vi "dataValueToXml.vi"(8 "error in (no error)":errorcluster, 11 "RampEvent in":refnum<class "RampEvent.lvclass">) -> (0 "error out":errorcluster, 2 "dataValueXml":refnum<class "xmlNode.lvclass">, 3 "RampEvent out":refnum<class "RampEvent.lvclass">)   [LabVIEW 2009, in "Tools.lvlib" / "Scripting.lvlib" / "RampEvent.lvclass"]
uses:
  RampEvent.lvclass
  xmlNode/xmlNode.lvclass
  DatabaseHelpers/Database Objects/Channel/Channel.lvclass
  ScriptEvent.lvclass
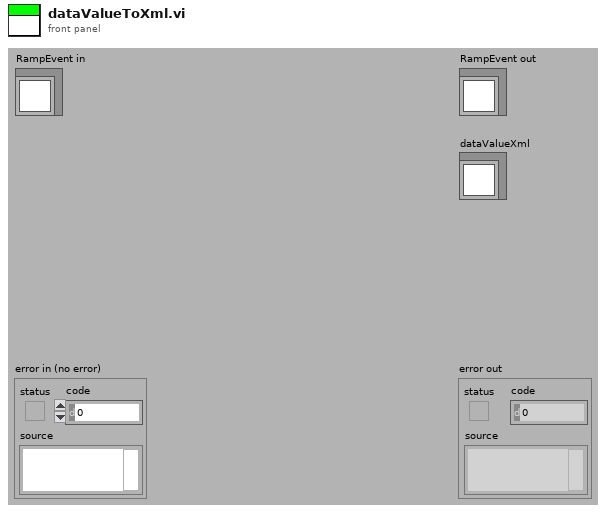
[diagram p1: front panel]
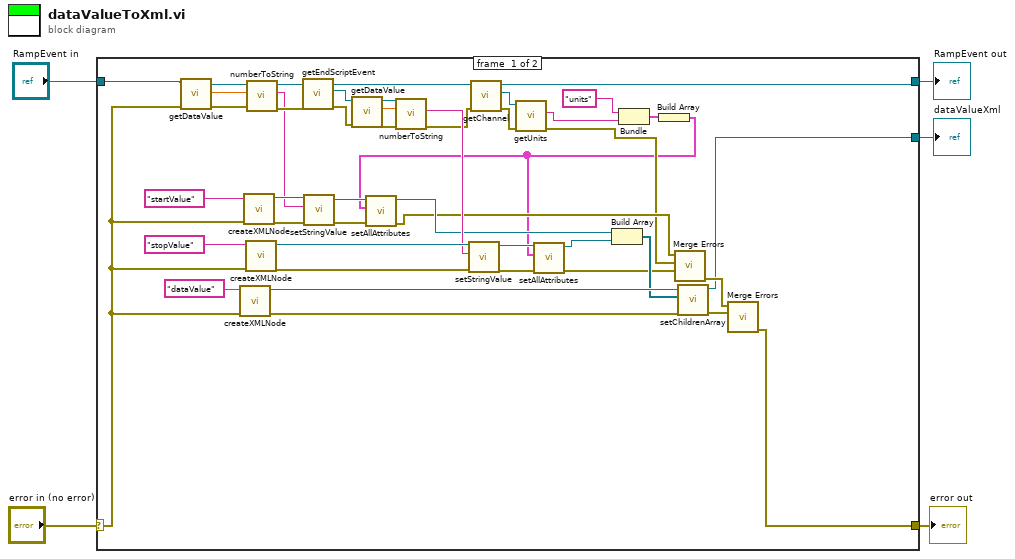
[diagram p0: block diagram]
diagram:
  n1 = case shown="No Error" "error in (no error)" {
    selector: "error in (no error)" -> [w7 w52]
    tunnel: [w6 w52] -> w4
    tunnel: "RampEvent in" -> [w39 w53]
    tunnel: [w9 w53] -> w2
    tunnel: [w8 _] -> w1
    frame #0 {
      n2 = call "getDataValue.vi"("error in (no error)"=w7, "ScriptEvent.lvclass in"=w39) -> ("error out"=w35:errorcluster, "dataValue"=w32:dbl, "ScriptEvent.lvclass out"=w36:refnum<class "RampEvent.lvclass">)  [unwired: 7 in]
      n3 = call "createXMLNode.vi"("error in (no error)"=w7, "name"="dataValue") -> ("error out"=w43:errorcluster, "xmlNode out"=w44:refnum<class "xmlNode.lvclass">)  [unwired: 8 in]
      n4 = call "createXMLNode.vi"("error in (no error)"=w7, "name"="startValue") -> ("error out"=w47:errorcluster, "xmlNode out"=w48:refnum<class "xmlNode.lvclass">)  [unwired: 8 in]
      n5 = call "createXMLNode.vi"("error in (no error)"=w7, "name"="stopValue") -> ("error out"=w45:errorcluster, "xmlNode out"=w46:refnum<class "xmlNode.lvclass">)  [unwired: 8 in]
      n6 = call "numberToString.vi"("error in (no error)"=w35, "Numeric"=w32, "ScriptEvent in"=w36) -> ("error out"=w34:errorcluster, "String"=w31:string, "ScriptEvent out"=w33:refnum<class "RampEvent.lvclass">)  [unwired: 6 in]
      n7 = call "getEndScriptEvent.vi"("error in (no error)"=w34, "RampEvent.lvclass in"=w33) -> ("error out"=w37:errorcluster, "ScriptEvent.lvclass"=w38:refnum<class "ScriptEvent.lvclass">, "RampEvent.lvclass out"=w25:refnum<class "RampEvent.lvclass">)  [unwired: 7 in]
      n8 = call-dynamic "setStringValue.vi"("error in (no error)"=w47, "stringValue"=w31, "xmlNode.lvclass in"=w48) -> ("error out"=w19:errorcluster, "xmlNode.lvclass out"=w18:refnum<class "xmlNode.lvclass">)  [unwired: 7 in]
      n9 = call "getDataValue.vi"("error in (no error)"=w37, "ScriptEvent.lvclass in"=w38) -> ("error out"=w29:errorcluster, "dataValue"=w28:dbl, "ScriptEvent.lvclass out"=w30:refnum<class "ScriptEvent.lvclass">)  [unwired: 7 in]
      n10 = call "numberToString.vi"("error in (no error)"=w29, "Numeric"=w28, "ScriptEvent in"=w30) -> ("error out"=w24:errorcluster, "String"=w27:string)  [unwired: 6 in, 1 out]
      n11 = call-dynamic "setStringValue.vi"("error in (no error)"=w45, "stringValue"=w27, "xmlNode.lvclass in"=w46) -> ("error out"=w13:errorcluster, "xmlNode.lvclass out"=w14:refnum<class "xmlNode.lvclass">)  [unwired: 7 in]
      n12 = call-dynamic "getChannel.vi"("error in (no error)"=w24, "ScriptEvent.lvclass in"=w25) -> ("error out"=w22:errorcluster, "Channel.lvclass"=w23:refnum<class "Channel.lvclass">, "ScriptEvent.lvclass out"=w9:refnum<class "RampEvent.lvclass">)  [unwired: 7 in]
      n13 = call-dynamic "getUnits.vi"("error in (no error)"=w22, "Channel.lvclass in"=w23) -> ("error out"=w15:errorcluster, "units"=w21:string)  [unwired: 7 in, 1 out]
      n14 = Bundle("units", "units"=w21) -> (w20:cluster{string, "units":string})  [unwired: 1 in]
      n15 = Build Array(w20) -> (w12:cluster{string, "units":string}[])
      n16 = call-dynamic "setAllAttributes.vi"("error in (no error)"=w19, "attributes"=w12, "xmlNode in"=w18) -> ("error out"=w16:errorcluster, "xmlNode out"=w17:refnum<class "xmlNode.lvclass">)  [unwired: 7 in]
      n17 = call-dynamic "setAllAttributes.vi"("error in (no error)"=w13, "attributes"=w12, "xmlNode in"=w14) -> ("error out"=w10:errorcluster, "xmlNode out"=w11:refnum<class "xmlNode.lvclass">)  [unwired: 7 in]
      n18 = Build Array(w17, w11) -> (w42:refnum<class "xmlNode.lvclass">[])
      n19 = call <vilib>:"Merge Errors.vi"("error in 3 (no error)"=w10, "error in 2 (no error)"=w15, "error in 1 (no error)"=w16) -> ("error out"=w41:errorcluster)  [unwired: 4 in]
      n20 = call-dynamic "setChildrenArray.vi"("error in (no error)"=w43, "Children"=w42, "xmlNode.lvclass in"=w44) -> ("error out"=w40:errorcluster, "xmlNode.lvclass out"=w8:refnum<class "xmlNode.lvclass">)  [unwired: 7 in]
      n21 = call <vilib>:"Merge Errors.vi"("error in 2 (no error)"=w40, "error in 1 (no error)"=w41) -> ("error out"=w6:errorcluster)  [unwired: 5 in]
    }
    frame #1 {
    }
  }
  "error out" <- w4
  "RampEvent out" <- w2
  "dataValueXml" <- w1
